vi "Verify a VI.vi"(8 "error in":errorcluster) -> (0 "error out":errorcluster)   [LabVIEW 2020, in "Caraya Extension Tests.lvclass"]
uses:
  Caraya Extension Tests.lvclass
  <vilib>/addons/_JKI Toolkits/Caraya/classes/Test/Test.lvclass
  Source/Extensions/Caraya.Extension/Caraya.Extension.lvlib
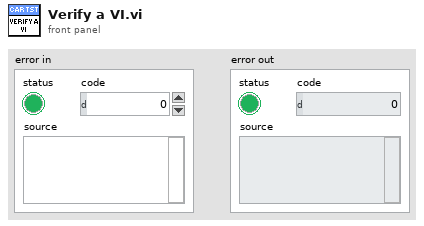
[diagram p1: front panel]
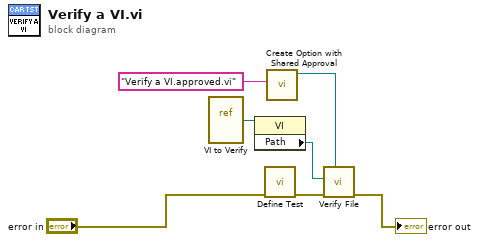
[diagram p0: block diagram]
diagram:
  n1 = vi-ref "VI to Verify.vi"() -> (w4:refnum<vi>)
  n2 = property on="Property Node" class="VI"(reference=w4) -> ("Path"=w3:path)  [unwired: 1 in, 2 out]
  n3 = call <vilib>:"Define Test.vi"("error in (no error)"="error in") -> ("error out"=w5:errorcluster)  [unwired: 9 in, 1 out]
  n4 = call "Create Option with Shared Approval.vi"("Filename"="Verify a VI.approved.vi") -> ("Options outs"=w1:refnum<class "Options.lvclass">)  [unwired: 10 in]
  n5 = call "Verify File.vi"("Options"=w1, "error in"=w5, "path to file"=w3) -> ("error out"=→"error out":errorcluster)  [unwired: 7 in, 1 out]
